vi "OnlyGetBmp_jpg_Img.vi"(0 "path":path) -> (1 "subarray":string[](array[string]), 2 "Array":path[](array[path]))   [LabVIEW 2014]
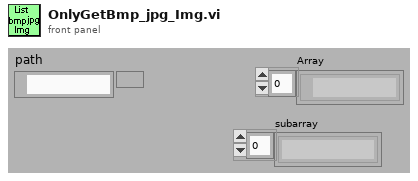
[diagram p1: front panel]
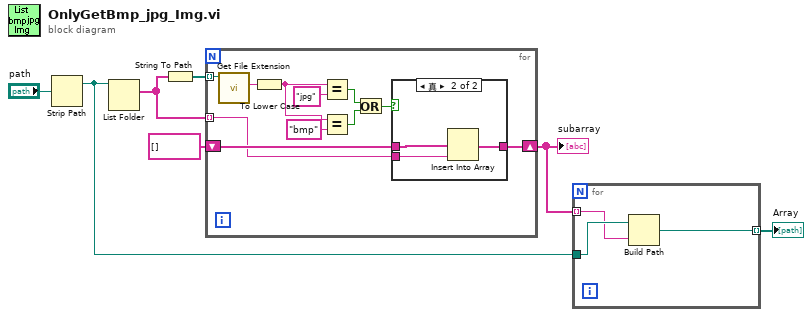
[diagram p0: block diagram]
diagram:
  n1 = Strip Path(path="path") -> (stripped path=w2:path)  [unwired: 1 out]
  n2 = List Folder(path=w2) -> (filenames=w4:string[])  [unwired: 1 in, 5 out]
  n3 = String To Path(string=w4) -> (path=w6:path[])
  n4 = for {
    tunnel: w6 -> [w18] mode=indexing
    shift-right: [w10] -> w3
    shift-left: string[] [] ("subarray") -> [w11]
    tunnel: w4 -> [w8] mode=indexing
    n5 = call <vilib>:"Get File Extension.vi"("file"=w18) -> ("lowercase file extension"=w17:string)  [unwired: 1 in, 9 out]
    n6 = To Lower Case(string=w17) -> (all lower case string=w9:string)
    n7 = Equal?(x=w9, y="jpg") -> (x = y?=w14:bool)
    n8 = Equal?(x=w9, y="bmp") -> (x = y?=w13:bool)
    n9 = Or(x=w14, y=w13) -> (x .or. y?=w12:bool)
    n10 = case shown="真" w12 {
      tunnel: w11 -> [w19 w22]
      tunnel: [w19 w20] -> w10
      tunnel: w8 -> [_ w21]
      frame False {
      }
      frame True {
        n11 = Insert Into Array(array=w22, new element=w21) -> (w20:string[])  [unwired: 1 in]
      }
    }
  }
  "subarray" <- w3
  n12 = for {
    tunnel: w3 -> [w24] mode=indexing
    tunnel: w2 -> [w25]
    tunnel: [w23] -> w1 mode=indexing
    n13 = Build Path(base path=w25, name or relative path=w24) -> (appended path=w23:path)
  }
  "Array" <- w1
